vi "run_tests.vi"(11 "Command Line":string[](array[string])) -> (2 "stdout | stderr":string, 3 "Return Code":i32)   [LabVIEW 2020]
uses:
  <vilib>/Utility/error.llb/DialogType.ctl
  20ab466a-1420-47d7-bd04-4ec556d045c0.vi
  <vilib>/Utility/error.llb/Error Cluster From Error Code.vi
  <vilib>/Comparison/Equal/Equal Functor/Equal Functor.lvclass
  <vilib>/ErrorRing/Error Ring.xnode
panel:
  out "Full Report":string
  out "All Tests Passed":bool
  out "error out":errorcluster
  # "Required by LabVIEWCLI\n(via connector pane)"
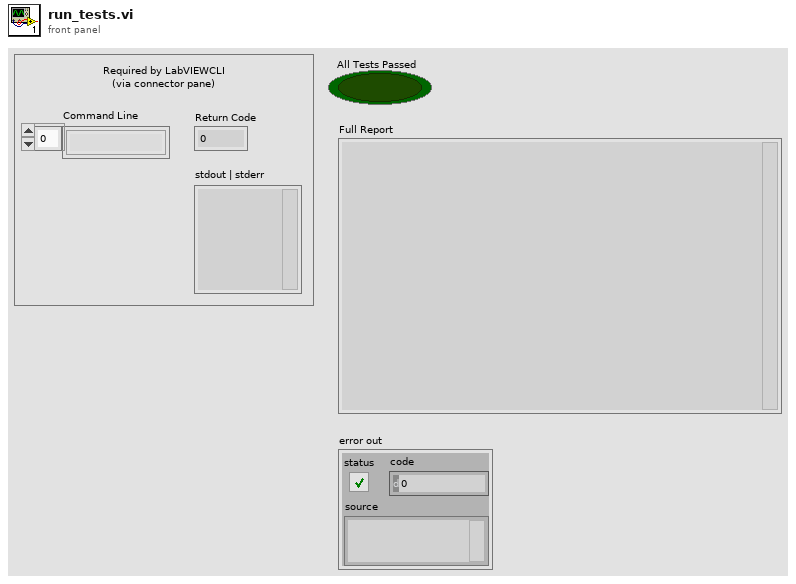
[diagram p1: front panel]
types:
  T1 = typedef "DialogType.ctl" = u16
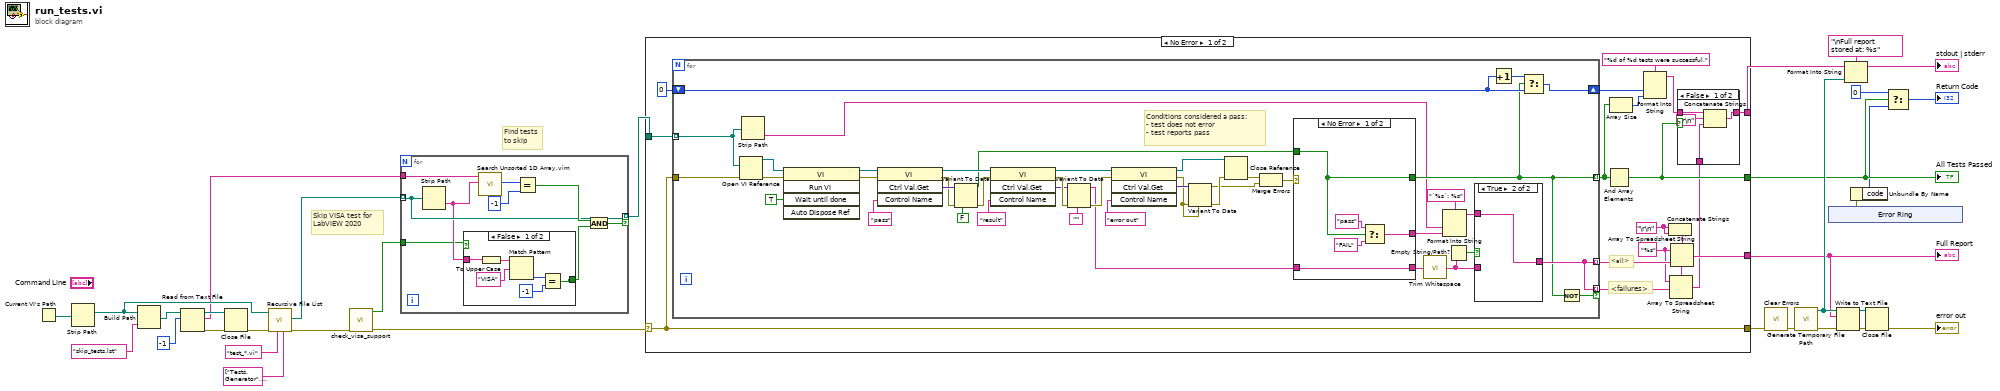
[diagram p0: block diagram]
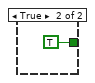
[diagram p2: hidden frame]
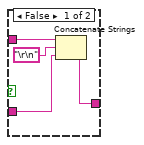
[diagram p4: hidden frame]
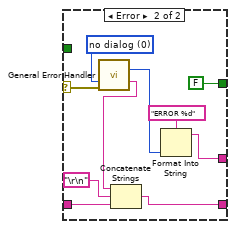
[diagram p5: hidden frame]
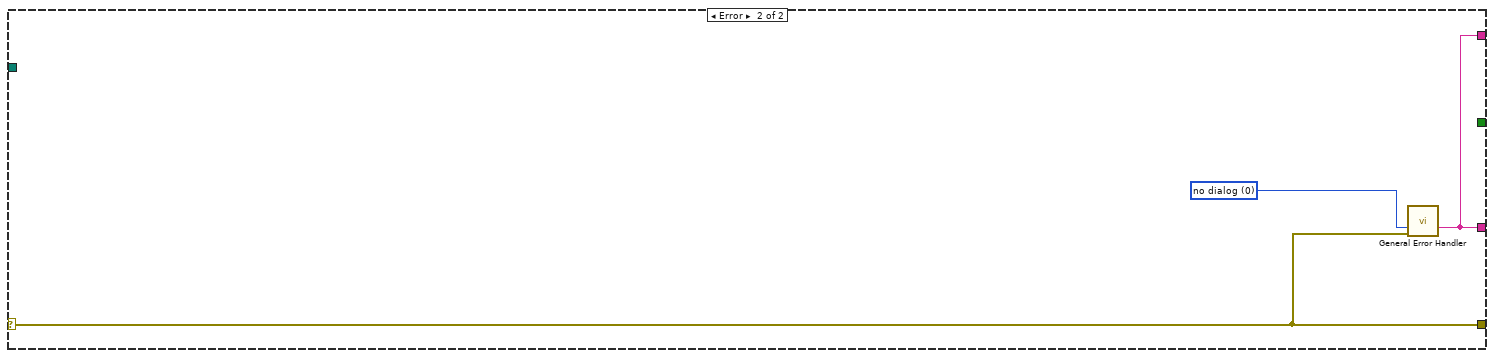
[diagram p6: hidden frame]
diagram:
  # "Skip VISA test for LabVIEW 2020"
  # "Find tests\nto skip"
  n1 = Current VI's Path() -> (path=w32:path)
  n2 = Strip Path(path=w32) -> (stripped path=w11:path)  [unwired: 1 out]
  n3 = Build Path(base path=w11, name or relative path="skip_tests.lst") -> (appended path=w9:path)
  n4 = Read from Text File(file (use dialog)=w9, count=-1) -> (refnum out=w12:refnum<file>, text=w6:string[], error out=w14:errorcluster)  [unwired: 2 in, 1 out]
  n5 = Close File(refnum=w12, error in=w14) -> (error out=w13:errorcluster)  [unwired: 1 out]
  n6 = call <vilib>:"Recursive File List.vi"("Folders to Exclude"=string[] ["Tests.Generator", "Measurement Server", "Pin Map Client", "Session Management Client"], "pattern"="test_*.vi", "error in (no error)"=w13, "Folder Path"=w11) -> ("error out"=w3:errorcluster, "All Files in Dir"=w7:path[])  [unwired: 3 in, 3 out]
  n7 = call "check_visa_support.vi"("error in"=w3) -> ("error out"=w2:errorcluster, "visa supported"=w4:bool)  [unwired: 9 in]
  n8 = for {
    tunnel: w7 -> [w36] mode=indexing
    tunnel: w6 -> [w41]
    tunnel: [w36] -> w5 mode=indexing if=w38
    tunnel: w4 -> [w33]
    n9 = Strip Path(path=w36) -> (name=w34:string)  [unwired: 1 out]
    n10 = case shown="False" w33 {
      tunnel: [w42 TRUE] -> w35
      tunnel: w34 -> [w43 _]
      frame False {
        n11 = To Upper Case(1:w43) -> (0:w47:string)
        n12 = Match Pattern(string=w47, regular expression="VISA") -> (offset past match=w46:i32)  [unwired: 1 in, 3 out]
        n13 = Equal?(x=w46, y=-1) -> (x = y?=w42:bool)
      }
      frame True {
      }
    }
    n14 = call "Search Unsorted 1D Array.vim"("element"=w34, "unsorted 1D array"=w41) -> ("index of element"=w40:i32)  [unwired: 9 in]
    n15 = Equal?(x=w40, y=-1) -> (x = y?=w39:bool)
    n16 = And(x=w39, y=w35) -> (x .and. y?=w38:bool)
  }
  n17 = case shown="No Error" w2 {
    selector: w2 -> [w64 w135]
    tunnel: w5 -> [w65 _]
    tunnel: [w64 w135] -> w30
    tunnel: [w57 _] -> w21
    tunnel: [w54 w133] -> w22
    tunnel: [w55 w133] -> w27
    frame No Error {
      w50 = "%s" ("format string")
      w63 = "\r\n"
      # "<failures>"
      # "<all>"
      n18 = for {
        tunnel: w65 -> [w72] mode=indexing
        tunnel: w64 -> [w112]
        tunnel: [w74] -> w59 mode=indexing
        tunnel: [w78] -> w53 mode=indexing
        tunnel: [w78] -> w52 mode=indexing if=w77
        shift-right: [w73] -> w60
        shift-left: 0 -> [w75]
        # "Conditions considered a pass:\n- test does not error\n- test reports pass"
        n19 = Open VI Reference(vi path=w72, error in (no error)=w112) -> (vi reference=w111:refnum<vi>, error out=w110:errorcluster)  [unwired: 4 in]
        n20 = Strip Path(path=w72) -> (name=w71:string)  [unwired: 1 out]
        n21 = invoke class="VI" method="Run VI"(reference=w111, error in=w110, "Wait until done"=TRUE ("Wait Until Done")) -> (reference out=w108:refnum<vi>, error out=w107:errorcluster)  [unwired: 2 in, 3 out]
        n22 = invoke class="VI" method="Ctrl Val.Get"(reference=w108, error in=w107, "Control Name"="pass") -> (reference out=w97:refnum<vi>, error out=w104:errorcluster, "Get Control Value Variant"=w105:variant)  [unwired: 1 in, 1 out]
        n23 = Variant To Data(error in=w104, type=FALSE, Variant=w105) -> (data=w86:bool, error out=w101:errorcluster)
        n24 = invoke class="VI" method="Ctrl Val.Get"(reference=w97, error in=w101, "Control Name"="result") -> (reference out=w92:refnum<vi>, error out=w102:errorcluster, "Get Control Value Variant"=w99:variant)  [unwired: 1 in, 1 out]
        n25 = Variant To Data(error in=w102, type="", Variant=w99) -> (data=w83:string, error out=w95:errorcluster)
        n26 = invoke class="VI" method="Ctrl Val.Get"(reference=w92, error in=w95, "Control Name"="error out") -> (reference out=w91:refnum<vi>, error out=w93:errorcluster, "Get Control Value Variant"=w96:variant)  [unwired: 1 in, 1 out]
        n27 = Variant To Data(error in=w93, type=w93, Variant=w96) -> (data=w88:errorcluster, error out=w94:errorcluster)
        n28 = Close Reference(reference=w91, error in (no error)=w94) -> (error out=w89:errorcluster)
        n29 = Merge Errors(w89, w88) -> (w87:errorcluster)
        n30 = case shown="No Error" w87 {
          selector: w87 -> [_ w130]
          tunnel: w86 -> [w120 _]
          tunnel: [w119 w127] -> w84
          tunnel: [w120 FALSE] -> w74
          tunnel: w83 -> [w118 w126]
          tunnel: [w118 w125] -> w82
          frame No Error {
            n31 = Select(t="pass" ("Control Name"), s=w120, f="FAIL" ("Control Name")) -> (s? t:f=w119:string)
          }
          frame Error {
            w131 = T1 0 items=["no dialog", "OK message", "continue or stop message", "OK message + warnings", "continue/stop + warnings"] ("type of dialog (OK msg:1)")
            n32 = call <vilib>:"General Error Handler.vi"("type of dialog (OK msg:1)"=w131, "error in (no error)"=w130) -> ("code out"=w129:i32, "message"=w124:string)  [unwired: 9 in, 3 out]
            n33 = Concatenate Strings(w124, "\r\n", w126) -> (w125:string)
            n34 = Format Into String(format string="ERROR %d", w129) -> (resulting string=w127:string)  [unwired: 2 in, 1 out]
          }
        }
        n35 = call <vilib>:"Trim Whitespace.vi"("string"=w82) -> ("trimmed string"=w81:string)  [unwired: 1 in]
        n36 = Format Into String(format string="`%s`: %s" ("Control Name"), w71, w84) -> (resulting string=w79:string)  [unwired: 2 in, 1 out]
        n37 = Empty String/Path?(string/path=w81) -> (empty?=w80:bool)
        n38 = case shown="True" w80 {
          tunnel: w81 -> [w115 _]
          tunnel: w79 -> [w116 w117]
          tunnel: [w114 w117] -> w78
          frame False {
            n39 = Concatenate Strings(w116, "\r\n", w115) -> (w114:string)
          }
          frame True {
          }
        }
        n40 = Increment(x=w75) -> (x+1=w76:i32)
        n41 = Select(t=w76, s=w74, f=w75) -> (s? t:f=w73:i32)
        n42 = Not(x=w74) -> (.not. x?=w77:bool)
      }
      n43 = And Array Elements(Boolean array=w59) -> (logical AND=w57:bool)
      n44 = Array Size(array=w59) -> (size(s)=w58:i32)
      n45 = Format Into String(format string="%d of %d tests were successful." ("Control Name"), w60, w58) -> (resulting string=w56:string)  [unwired: 2 in, 1 out]
      n46 = Concatenate Strings(w63, w63) -> (w51:string)
      n47 = Array To Spreadsheet String(delimiter (Tab)=w51, array=w52, 3:w50) -> (spreadsheet string=w49:string)
      n48 = Array To Spreadsheet String(delimiter (Tab)=w51, array=w53, 3:w50) -> (spreadsheet string=w54:string)
      n49 = case shown="False" w57 {
        tunnel: w56 -> [w69 w70]
        tunnel: [w66 w70] -> w55
        tunnel: w49 -> [w67 _]
        frame False {
          n50 = Concatenate Strings(w69, "\r\n", w67) -> (w66:string)
        }
        frame True {
        }
      }
    }
    frame Error {
      w134 = T1 0 items=["no dialog", "OK message", "continue or stop message", "OK message + warnings", "continue/stop + warnings"] ("type of dialog (OK msg:1)")
      n51 = call <vilib>:"General Error Handler.vi"("type of dialog (OK msg:1)"=w134, "error in (no error)"=w135) -> ("message"=w133:string)  [unwired: 9 in, 4 out]
    }
  }
  "All Tests Passed" <- w21
  "Full Report" <- w22
  n52 = call <vilib>:"Clear Errors.vi"("error in (no error)"=w30) -> ("error out"=w29:errorcluster)  [unwired: 5 in, 1 out]
  n53 = call <vilib>:"Generate Temporary File Path.vi"("error in (no error)"=w29) -> ("error out"=w24:errorcluster, "Unique Temporary File Path"=w25:path)  [unwired: 9 in]
  n54 = xnode "Error Ring"() -> ("error out"=w16:errorcluster)
  n55 = Write to Text File(file (use dialog)=w25, text=w22, error in=w24) -> (refnum out=w26:refnum<file>, error out=w23:errorcluster)  [unwired: 1 in, 1 out]
  n56 = Format Into String(format string="\nFull report stored at: %s" ("Control Name"), initial string=w27, w25) -> (resulting string=→"stdout | stderr":string)  [unwired: 1 in, 1 out]
  n57 = Unbundle By Name(w16) -> ("code"=w15:i32)
  n58 = Close File(refnum=w26, error in=w23) -> (error out=→"error out":errorcluster)  [unwired: 1 out]
  n59 = Select(t=0, s=w21, f=w15) -> (s? t:f=→"Return Code":i32)
